vi "image_processing.vi"(5 "NG_rules":T3, 7 "parameter":T2={"image imshow"=FALSE, "side length (mm)"=0.0, "side width (mm)"=0.0, "Main Range (Threshold)"={"Lower value"=73.0, "Upper value"=255.0}, "side velocity threshold"=0.0, "Sub Range (Threshold)"={"Lower value"=73.0, "Upper value"=255.0}, "close kernel size"=0.0, "open kernel size"=0.0, "side angle offest (threshold)"=0.0}, 11 "image":T1(plugin-control)) -> (0 "PASS":bool, 2 "NG code":dbl, 3 "display image":T1(plugin-control), 4 "angle offset":dbl)   [LabVIEW 2017]
uses:
  <vilib>/vision/NI_Vision_Development_Module.lvlib
panel:
  out "side width (mm)":dbl
  out "slope array":dbl[](array[numeric])
  out "max length ratio":dbl
  out "display image 3":T1(plugin-control)
  out "display image 2":T1(plugin-control)
  out "side angle offest":dbl
  out "side length (mm)":dbl
  out "ratio (cutting offest)":dbl
  out "damaged (mil)":dbl
  out "glitch (mil)":dbl
  out "open kernel size":dbl
  out "close kernel size":dbl
  in  "side velocity threshold":dbl
  out "Main Range (Threshold)":cluster{"Lower value":sgl, "Upper value":sgl}={"Lower value"=73.0, "Upper value"=255.0}
  out "image imshow":bool
  out "time image processing":u32
  out "time load image":u32
  out "Y Resolution":i32
  out "X Resolution":i32
  out "black image":T1(plugin-control)
  out "buffer image":T1(plugin-control)
  out "Sub Range (Threshold)":cluster{"Lower value":sgl, "Upper value":sgl}={"Lower value"=73.0, "Upper value"=255.0}
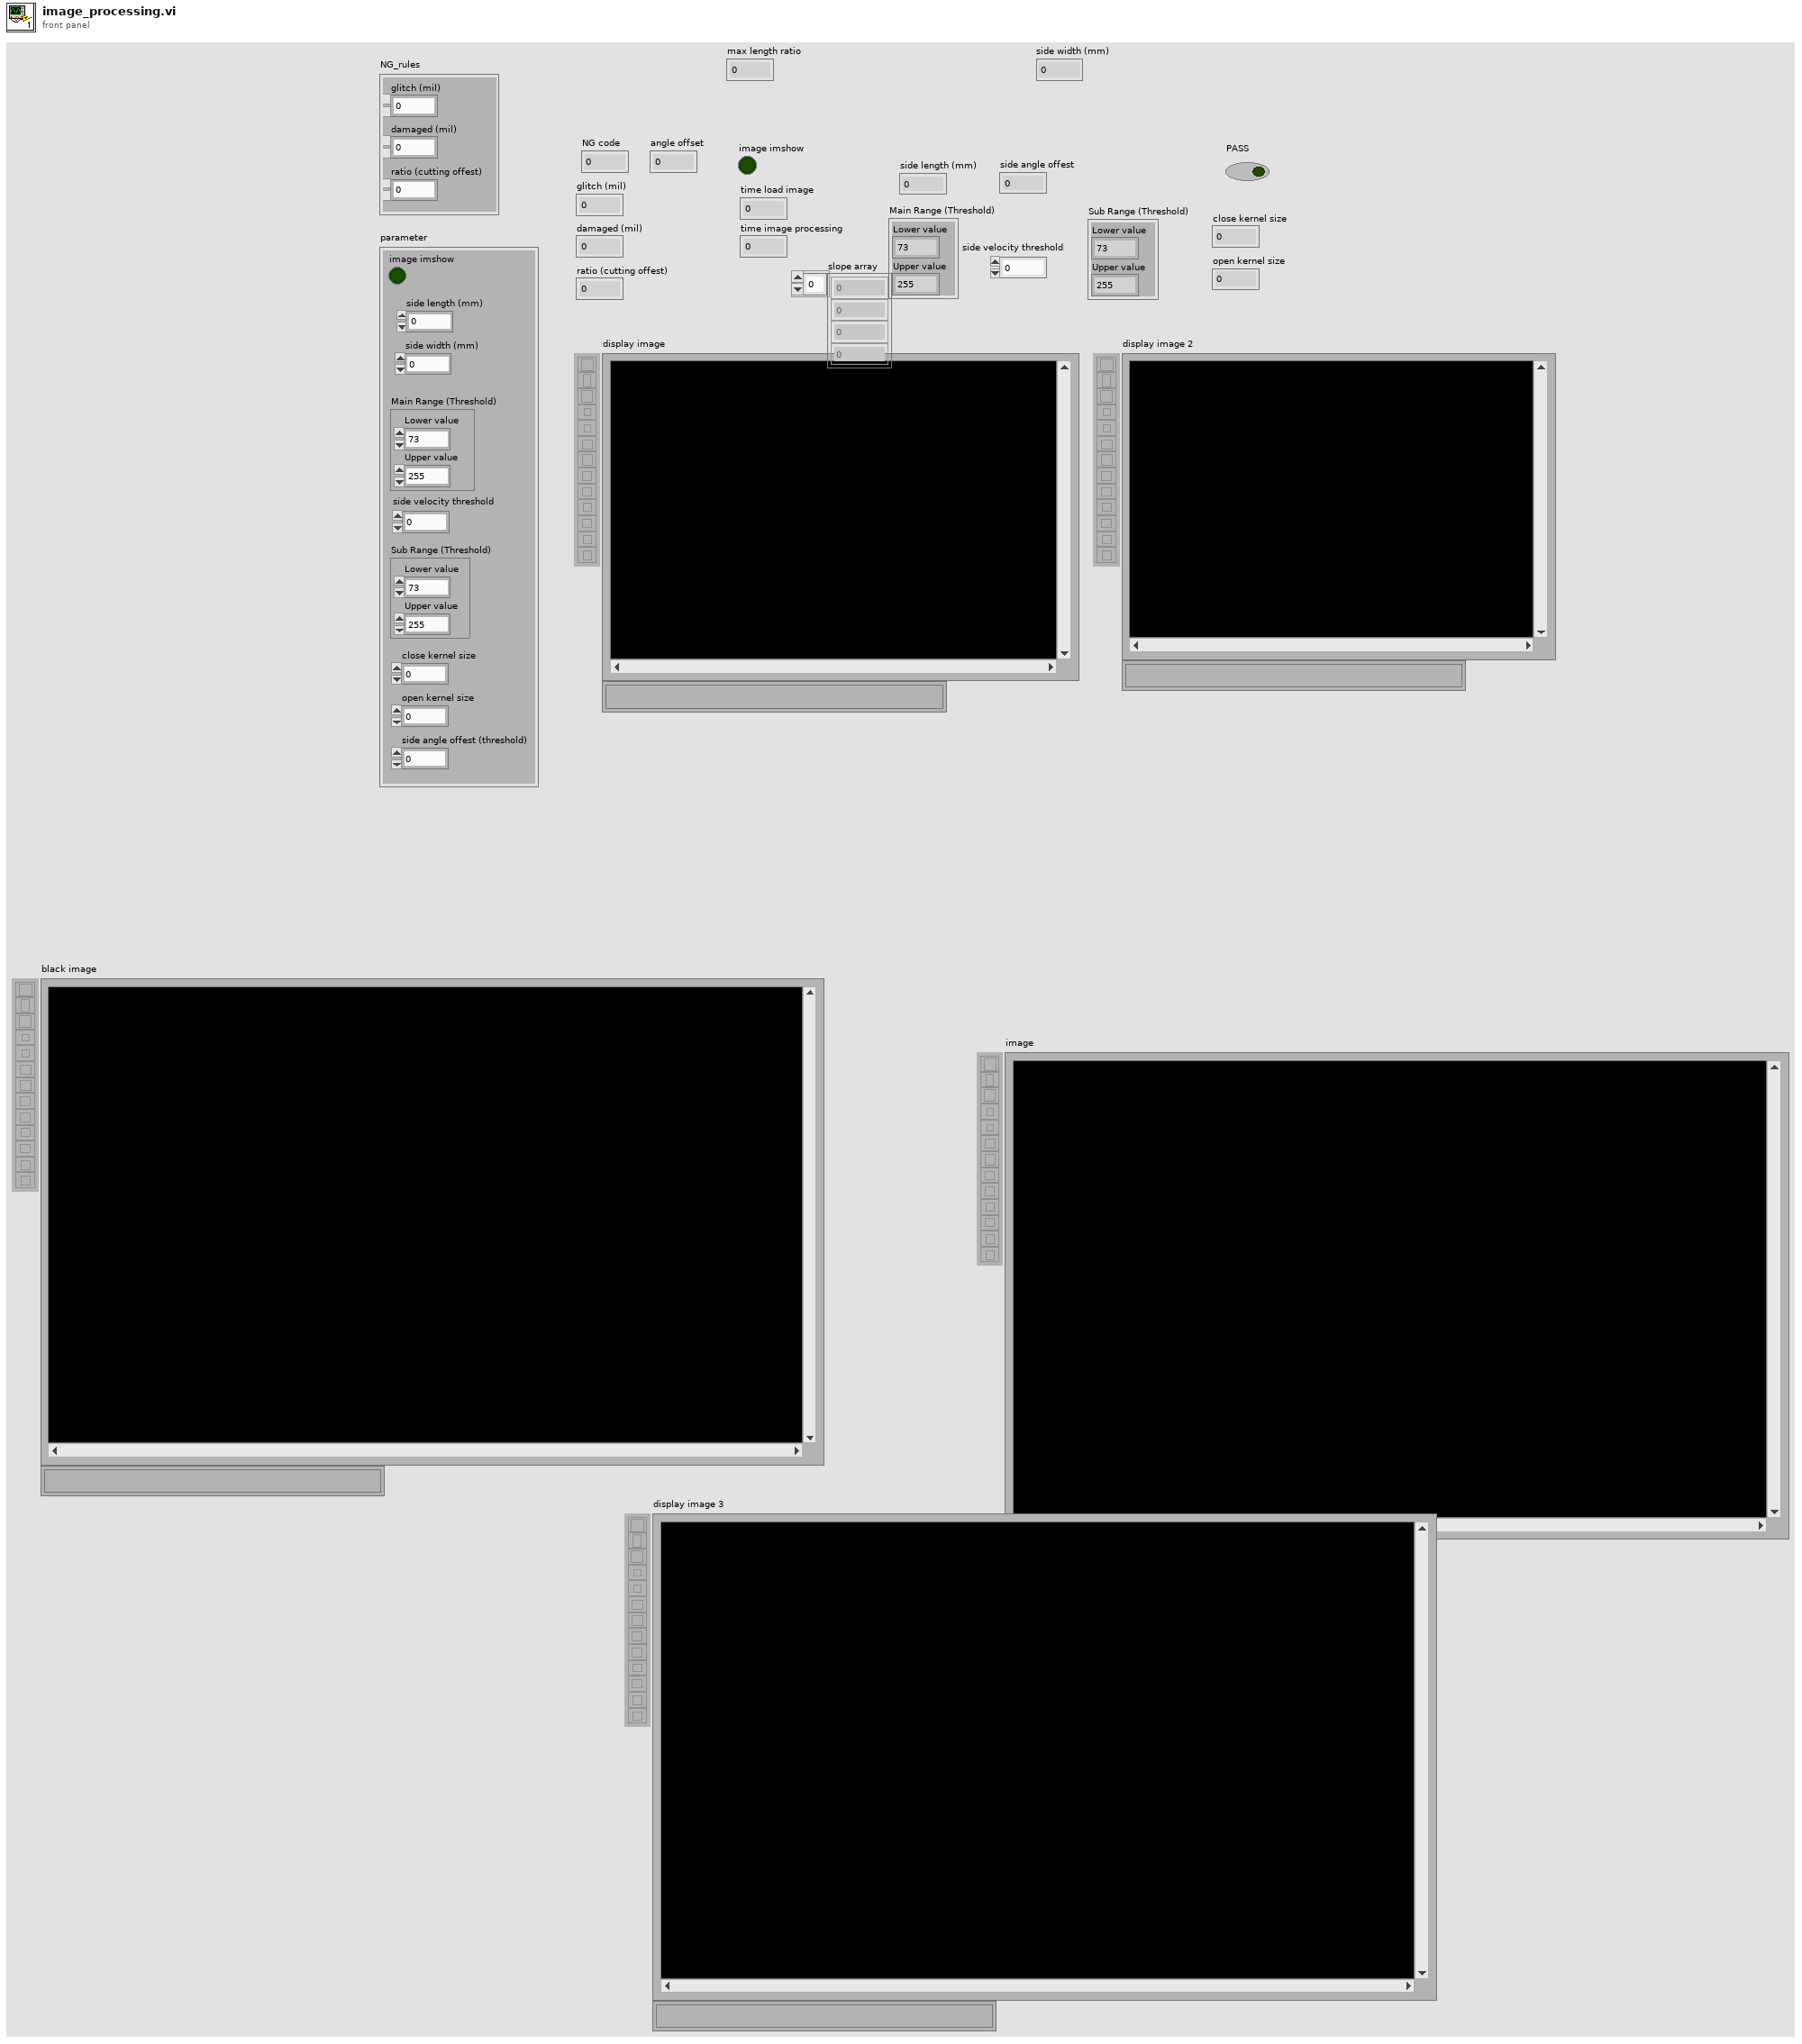
[diagram p1: front panel]
types:
  T1 = typedef "IMAQ Image.ctl" = refnum<image>
  T2 = cluster{"image imshow":bool, "side length (mm)":dbl, "side width (mm)":dbl, "Main Range (Threshold)":cluster{"Lower value":sgl, "Upper value":sgl}, "side velocity threshold":dbl, "Sub Range (Threshold)":cluster{"Lower value":sgl, "Upper value":sgl}, "close kernel size":dbl, "open kernel size":dbl, "side angle offest (threshold)":dbl}
  T3 = cluster{"glitch (mil)":dbl, "damaged (mil)":dbl, "ratio (cutting offest)":dbl}
  T4 = cluster{"Desired Font (Application)":enum16{"User-specified Font", "Application Font", "System Font", "Dialog Font"}, "[User-specified Font]":cluster{"Font Name":string, "Size":i16, "Strikeout?":bool, "Italic?":bool, "Underline?":bool, "Outline?":bool, "Shadow?":bool, "Bold?":bool, "Rotation Angle":dbl}, "Horizontal Alignment":i16, "Vertical Alignment":i16}
  T5 = enum32{"AutoM", "Close", "Dilate", "Erode", "Gradient", "Gradient out", "Gradient in", "Hit miss", "Open", "PClose", "POpen", "Thick", "Thin"}
  T6 = cluster{"Sigma":sgl, "HThresh":sgl, "LThres":sgl, "WindowSize":i32}
  T7 = cluster{"Number of Points":i32, "Open/Closed":i32, "Weight":dbl, "Contour Points":cluster{"X":dbl, "Y":dbl, "Curvature":dbl, "X Displacement":dbl, "Y Displacement":dbl}[]}[]
  T8 = cluster{"Left":i32, "Top":i32, "Right":i32, "Bottom":i32}
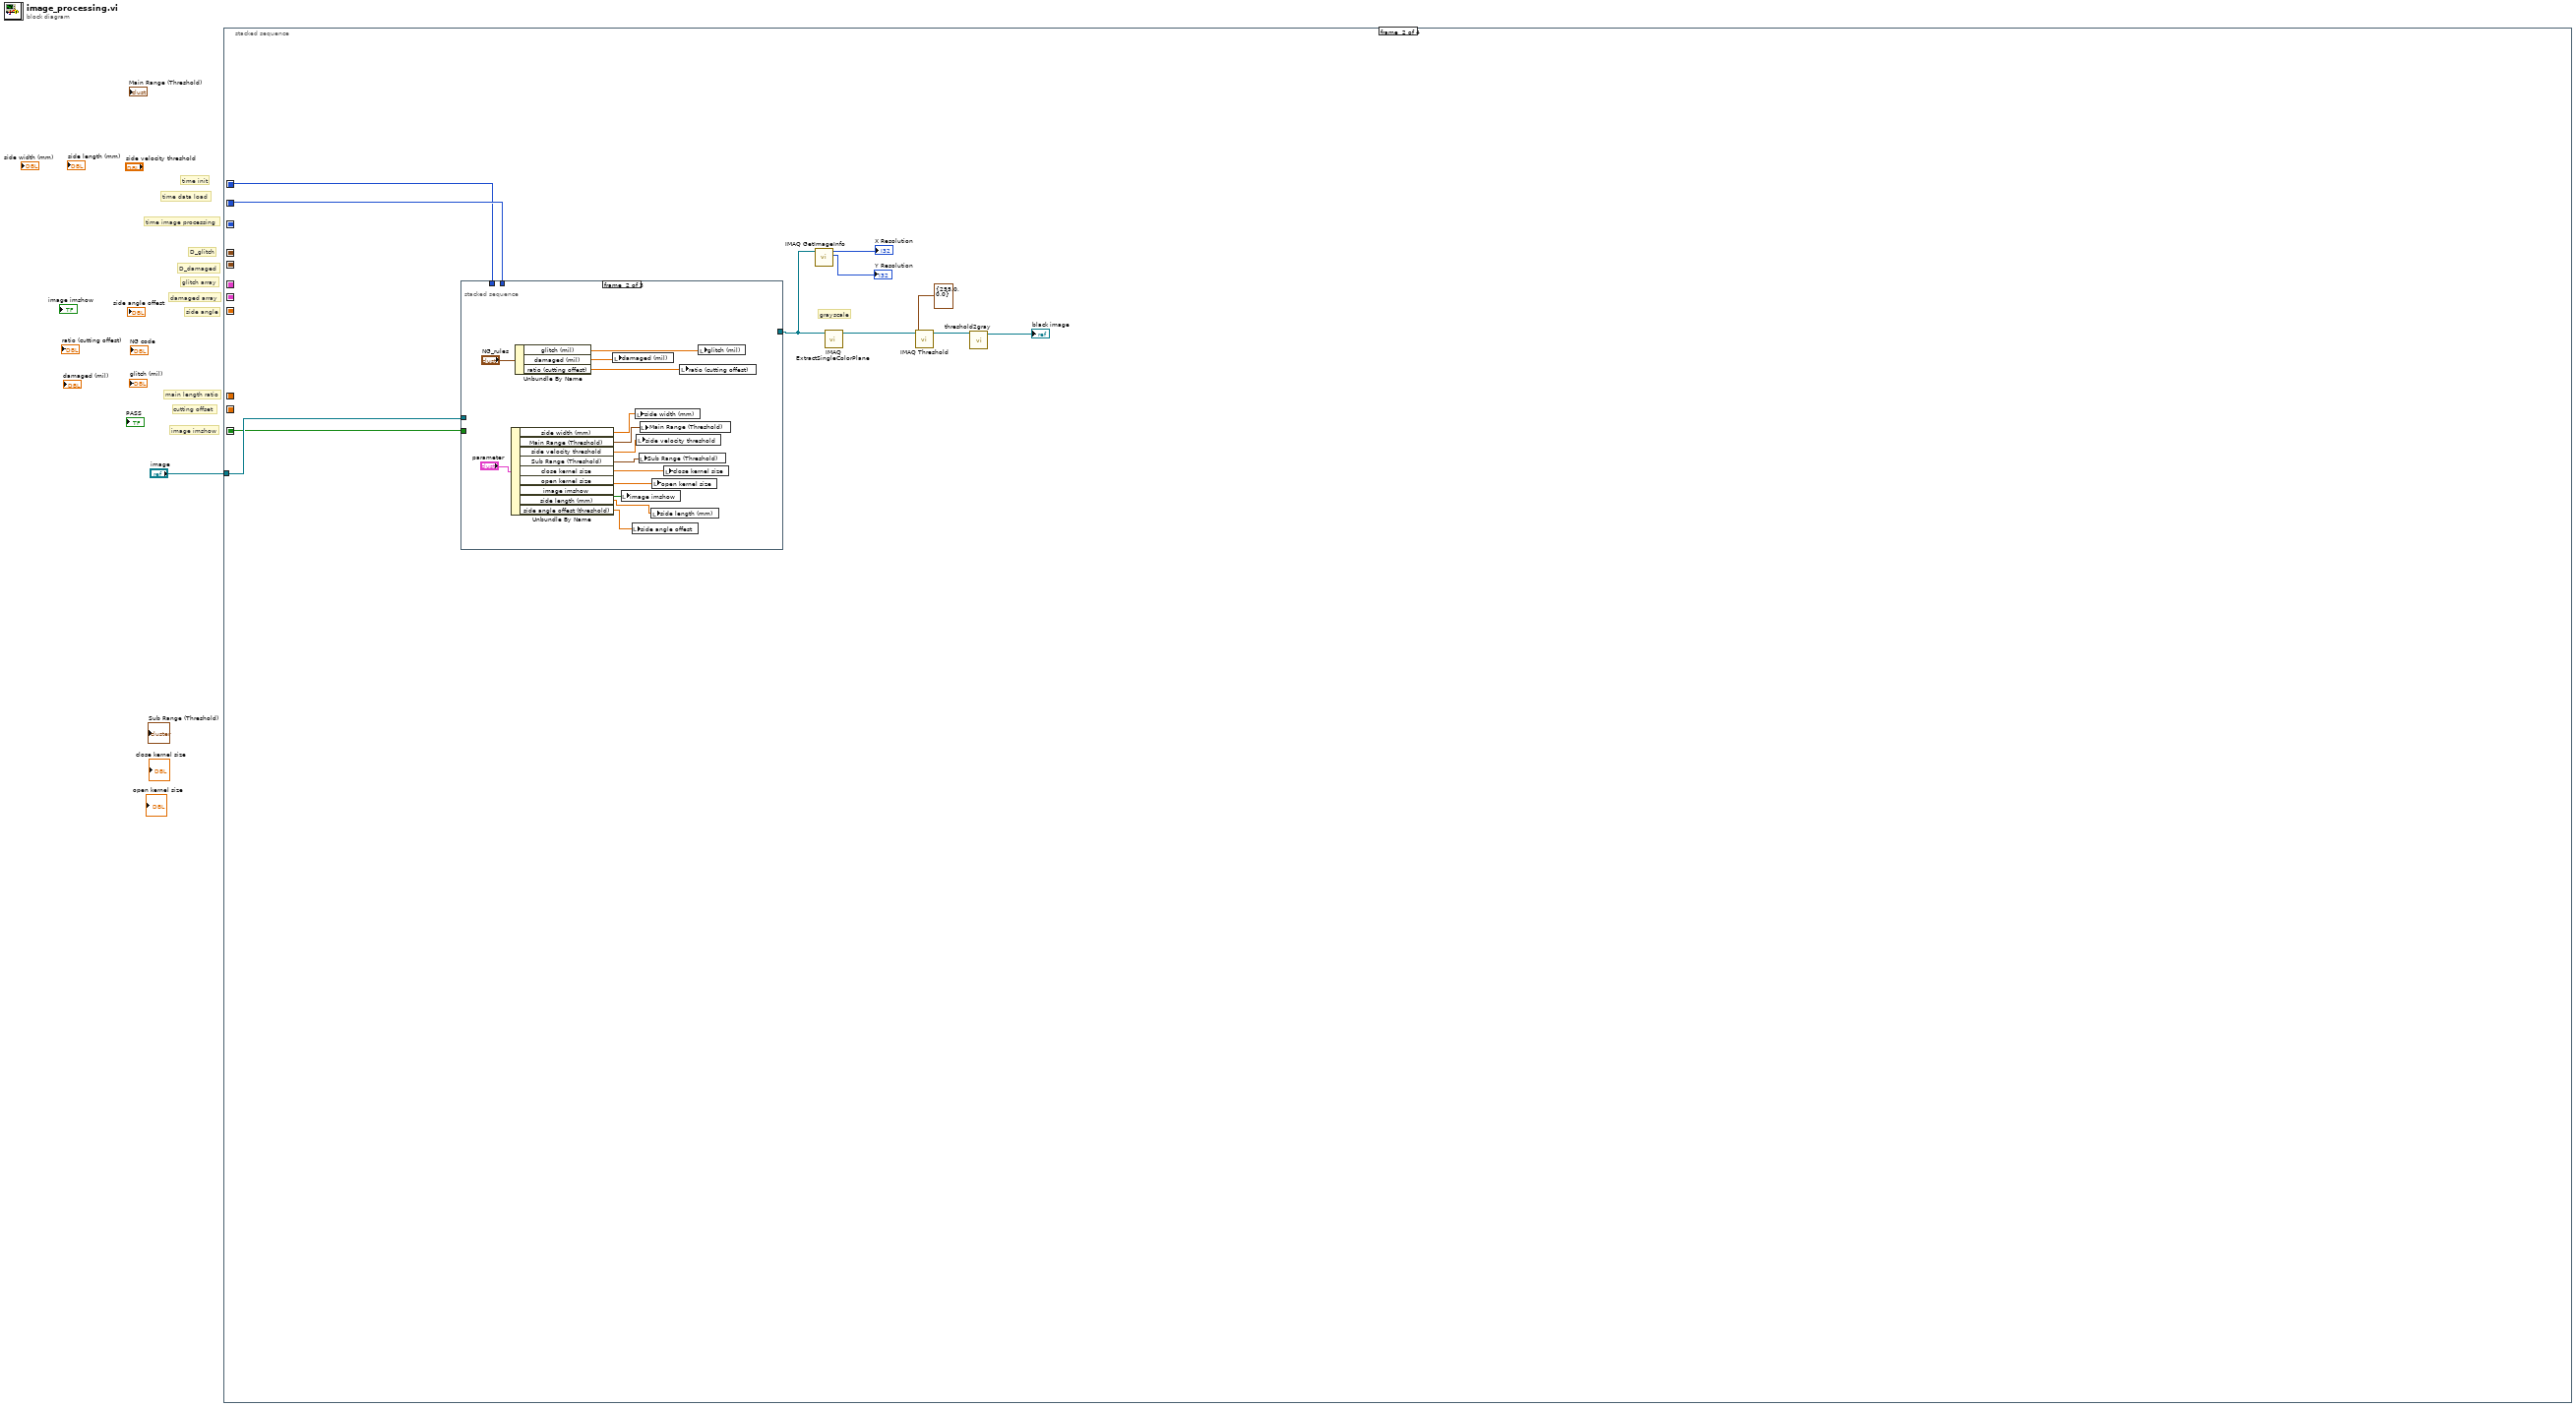
[diagram p0: block diagram]
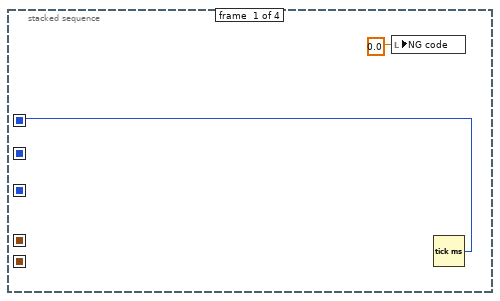
[diagram p2: hidden frame]
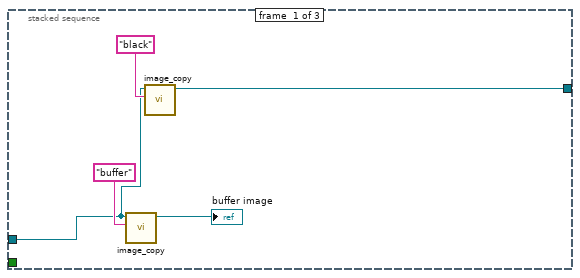
[diagram p3: hidden frame]
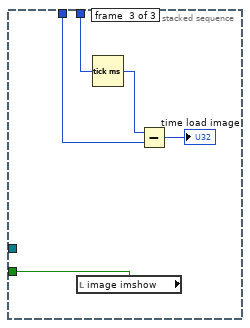
[diagram p4: hidden frame]
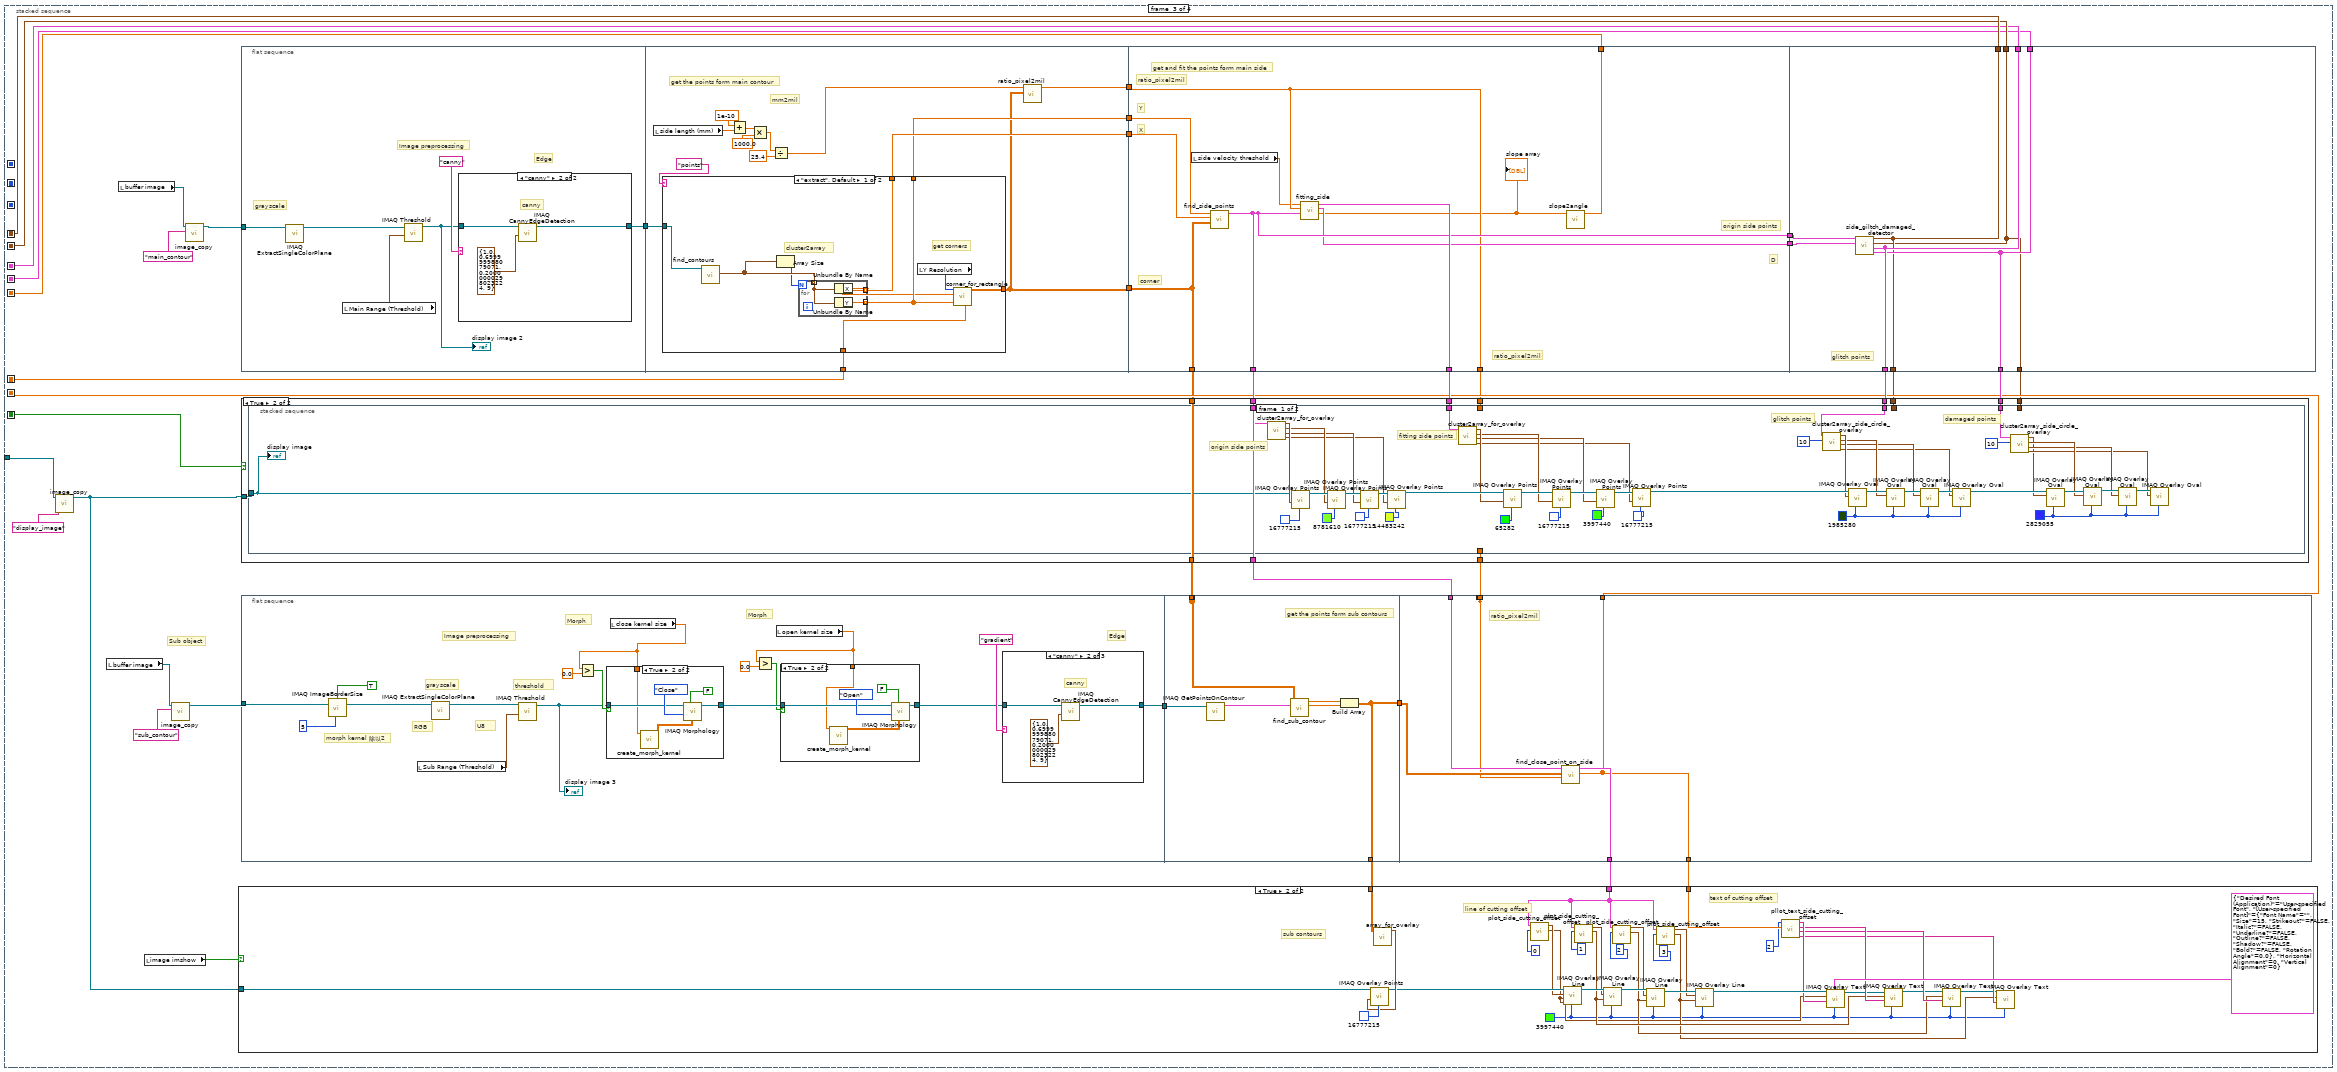
[diagram p5: hidden frame]
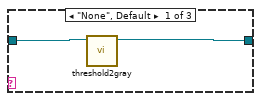
[diagram p9: hidden frame]
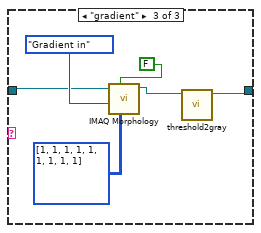
[diagram p10: hidden frame]
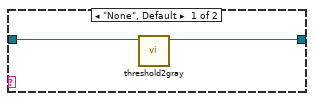
[diagram p11: hidden frame]
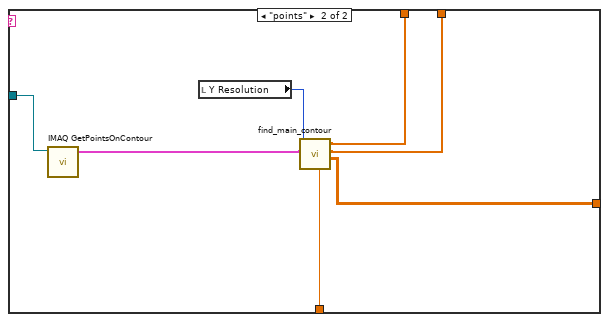
[diagram p12: hidden frame]
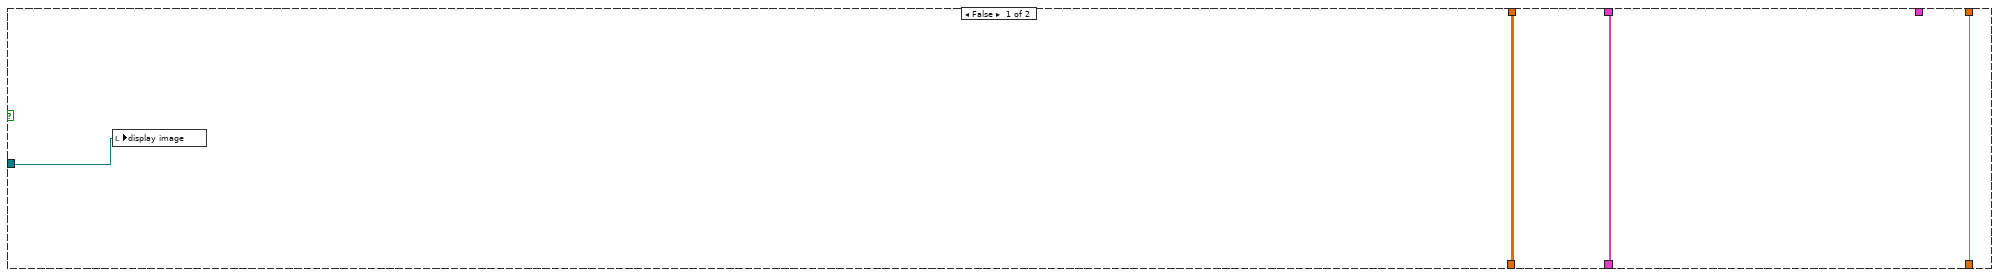
[diagram p13: hidden frame]
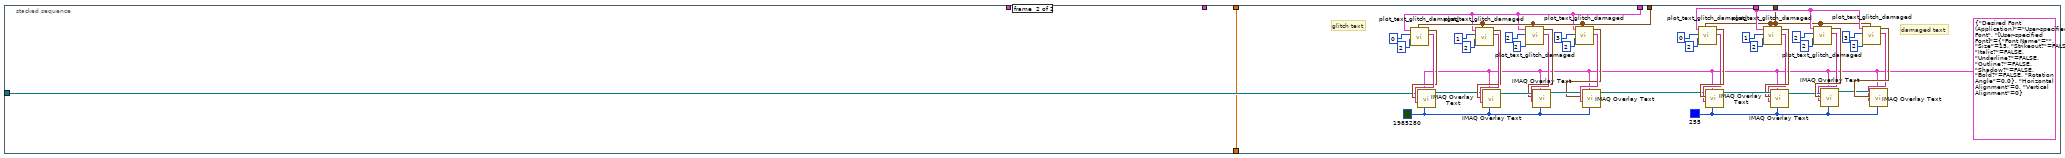
[diagram p14: hidden frame]
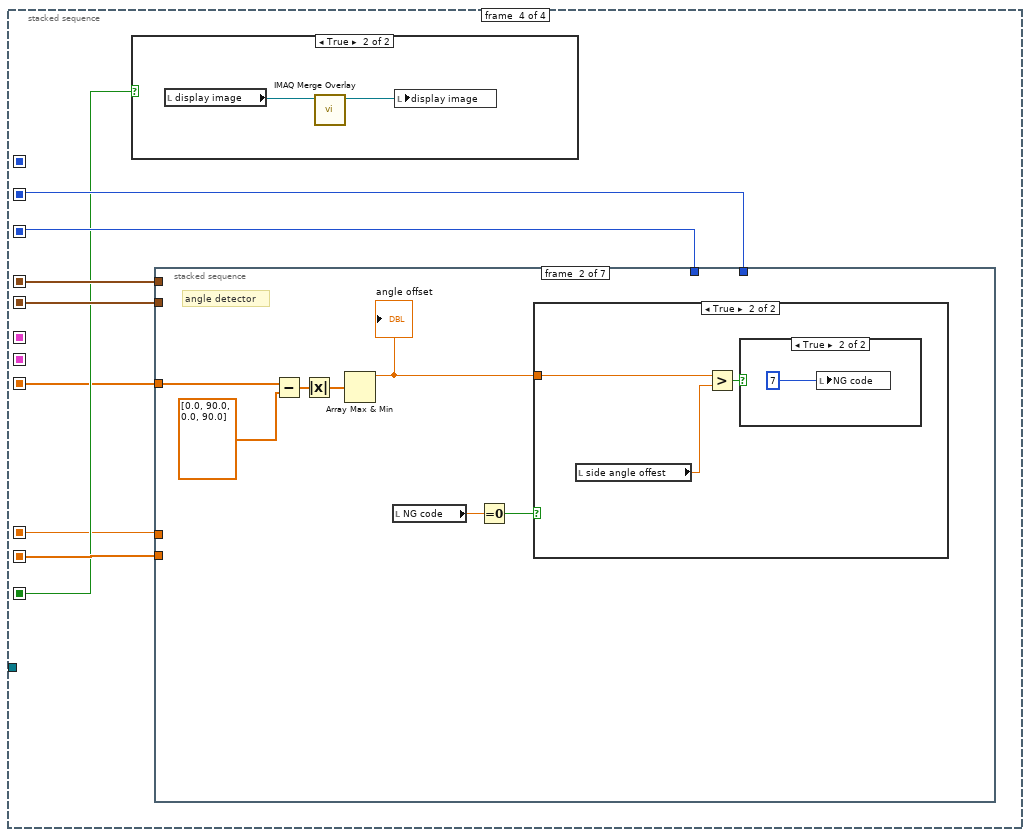
[diagram p15: hidden frame]
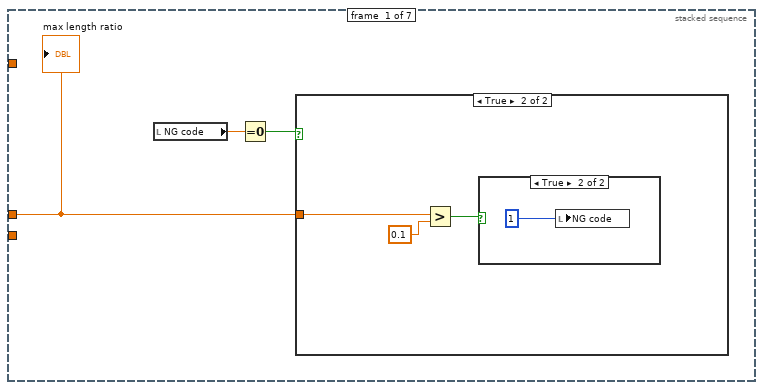
[diagram p17: hidden frame]
diagram:
  # "main length ratio"
  # "side angle"
  # "image imshow"
  # "cutting offset"
  # "damaged array"
  # "glitch array"
  # "D_damaged"
  # "D_glitch"
  # "time image processing"
  # "time data load"
  # "time init"
  n1 = stacked-sequence {
    seq-local: [w3 _ _ _] -> [_ w7 _ _]
    seq-local: [_ w8 _ _] -> [_ _ _ w340]
    seq-local: [_ _ _ w341] -> [_ _ _ _]
    seq-local: [_ _ w53 _] -> [_ _ _ w339]
    seq-local: [_ _ w52 _] -> [_ _ _ w338]
    seq-local: [_ _ w51 _] -> [_ _ _ _]
    seq-local: [_ _ w50 _] -> [_ _ _ _]
    seq-local: [_ _ w48 _] -> [_ _ _ w337]
    seq-local: [_ w4 _ _] -> [_ _ w42 w336]
    seq-local: [_ _ w41 _] -> [_ _ _ w335]
    seq-local: [_ _ w38 _] -> [_ _ _ w334]
    tunnel: "image" -> [_ w9 w60 _]
    frame #0 {
      n2 = local write "NG code"(0.0 ("NG code")) -> ()
      n3 = Tick Count (ms)() -> (millisecond timer value=w3:u32)
    }
    frame #1 {
      # "grayscale"
      n4 = stacked-sequence {
        tunnel: [w17 _ _] -> w12
        tunnel: w9 -> [w16 _ _]
        tunnel: [_ _ w37] -> w8
        tunnel: w7 -> [_ _ w36]
        tunnel: [_ _ w34] -> w4
        frame #0 {
          n5 = call "image_copy.vi"("buffer name"="buffer" ("Image Name"), "image in"=w16) -> ("imgae out"=→"buffer image":T1)  [unwired: 9 in]
          n6 = call "image_copy.vi"("buffer name"="black" ("Image Name"), "image in"=w16) -> ("imgae out"=w17:T1)  [unwired: 9 in]
        }
        frame #1 {
          n7 = Unbundle By Name("parameter") -> ("side width (mm)"=w20:dbl, "Main Range (Threshold)"=w28:cluster{"Lower value":sgl, "Upper value":sgl}, "side velocity threshold"=w27:dbl, "Sub Range (Threshold)"=w26:cluster{"Lower value":sgl, "Upper value":sgl}, "close kernel size"=w25:dbl, "open kernel size"=w24:dbl, "image imshow"=w23:bool, "side length (mm)"=w22:dbl, "side angle offest (threshold)"=w21:dbl)
          n8 = Unbundle By Name("NG_rules") -> ("glitch (mil)"=w32:dbl, "damaged (mil)"=w31:dbl, "ratio (cutting offest)"=w30:dbl)
          n9 = local write "damaged (mil)"(w31) -> ()
          n10 = local write "image imshow"(w23) -> ()
          n11 = local write "side angle offest"(w21) -> ()
          n12 = local write "side width (mm)"(w20) -> ()
          n13 = local write "side velocity threshold"(w27) -> ()
          n14 = local write "Sub Range (Threshold)"(w26) -> ()
          n15 = local write "Main Range (Threshold)"(w28) -> ()
          n16 = local write "side length (mm)"(w22) -> ()
          n17 = local write "open kernel size"(w24) -> ()
          n18 = local write "close kernel size"(w25) -> ()
          n19 = local write "ratio (cutting offest)"(w30) -> ()
          n20 = local write "glitch (mil)"(w32) -> ()
        }
        frame #2 {
          n21 = local read "image imshow"() -> (w34:bool)
          n22 = Tick Count (ms)() -> (millisecond timer value=w37:u32)
          n23 = Subtract(x=w37, y=w36) -> (x-y=→"time load image":u32)
        }
      }
      n24 = call "IMAQ GetImageInfo"("Image"=w12) -> ("Y Resolution"=→"Y Resolution":i32, "X Resolution"=→"X Resolution":i32)  [unwired: 3 in, 6 out]
      n25 = call "IMAQ ExtractSingleColorPlane"("Image Src"=w12) -> ("Image Dst Out"=w14:T1)  [unwired: 3 in, 7 out]
      n26 = call "IMAQ Threshold"("Range"=cluster{"Lower value":sgl, "Upper value":sgl} {"Lower value"=255.0, "Upper value"=0.0}, "Image Src"=w14) -> ("Image Dst Out"=w6:T1)  [unwired: 4 in, 5 out]
      n27 = call "threshold2gray.vi"("threshold image"=w6) -> ("grayscale image"=→"black image":T1)  [unwired: 10 in]
    }
    frame #2 {
      # "Sub object"
      n28 = call "image_copy.vi"("buffer name"="display_image" ("Image Name"), "image in"=w60) -> ("imgae out"=w59:T1)  [unwired: 9 in]
      n29 = local read "buffer image"() -> (w69:T1)
      n30 = local read "buffer image"() -> (w77:T1)
      n31 = local read "image imshow"() -> (w56:bool)
      n32 = call "image_copy.vi"("buffer name"="sub_contour" ("Image Name"), "image in"=w69) -> ("imgae out"=w68:T1)  [unwired: 9 in]
      n33 = call "image_copy.vi"("buffer name"="main_contour" ("Image Name"), "image in"=w77) -> ("imgae out"=w76:T1)  [unwired: 9 in]
      n34 = case shown="True" w56 {
        tunnel: w59 -> [_ w79]
        tunnel: w58 -> [_ w109]
        tunnel: w57 -> [_ w101]
        tunnel: w47 -> [_ w94]
        frame False {
        }
        frame True {
          w80 = u32 3997440 ("Text Color (black)")
          # "text of cutting offset"
          # "line of cutting offset"
          # "sub contours"
          n35 = call "array_for_overlay.vi"("Array in"=w109) -> ("Array out"=w110:cluster{"X":i32, "Y":i32}[])  [unwired: 10 in]
          n36 = call "IMAQ Overlay Points"("Color"=u32 16777215, "Array of Points"=w110, "Image"=w79) -> ("Image Out"=w108:T1)  [unwired: 7 in, 1 out]
          n37 = call "plot_side_cutting_offset.vi"("index"=0, "coord cluster"=w101) -> ("End Point out"=w81:cluster{"X":i32, "Y":i32}, "Start Point out"=w91:cluster{"X":i32, "Y":i32})  [unwired: 8 in]
          n38 = call "IMAQ Overlay Line"("Color"=w80, "End Point"=w81, "Start Point"=w91, "Image"=w108) -> ("Image Out"=w107:T1)  [unwired: 6 in, 1 out]
          n39 = call "plot_side_cutting_offset.vi"("index"=1, "coord cluster"=w101) -> ("End Point out"=w84:cluster{"X":i32, "Y":i32}, "Start Point out"=w96:cluster{"X":i32, "Y":i32})  [unwired: 8 in]
          n40 = call "IMAQ Overlay Line"("Color"=w80, "End Point"=w84, "Start Point"=w96, "Image"=w107) -> ("Image Out"=w106:T1)  [unwired: 6 in, 1 out]
          n41 = call "plot_side_cutting_offset.vi"("index"=2, "coord cluster"=w101) -> ("End Point out"=w83:cluster{"X":i32, "Y":i32}, "Start Point out"=w97:cluster{"X":i32, "Y":i32})  [unwired: 8 in]
          n42 = call "IMAQ Overlay Line"("Color"=w80, "End Point"=w83, "Start Point"=w97, "Image"=w106) -> ("Image Out"=w105:T1)  [unwired: 6 in, 1 out]
          n43 = call "plot_side_cutting_offset.vi"("index"=3, "coord cluster"=w101) -> ("End Point out"=w82:cluster{"X":i32, "Y":i32}, "Start Point out"=w98:cluster{"X":i32, "Y":i32})  [unwired: 8 in]
          n44 = call "IMAQ Overlay Line"("Color"=w80, "End Point"=w82, "Start Point"=w98, "Image"=w105) -> ("Image Out"=w99:T1)  [unwired: 6 in, 1 out]
          n45 = call "pllot_text_side_cutting_offset.vi"("D cutting offset array"=w94, "precision"=2 ("index")) -> ("Left side length"=w88:string, "Bottom side length"=w89:string, "Right side length"=w90:string, "Top side length"=w92:string)  [unwired: 6 in]
          n46 = call "IMAQ Overlay Text"("Text Color (black)"=w80, "Font, Size & Style"=T4 {"Desired Font (Application)"=enum."User-specified Font", "[User-specified Font]"={"Font Name"="", "Size"=15, "Strikeout?"=FALSE, "Italic?"=FALSE, "Underline?"=FALSE, "Outline?"=FALSE, "Shadow?"=FALSE, "Bold?"=FALSE, "Rotation Angle"=0.0}, "Horizontal Alignment"=0, "Vertical Alignment"=0}, "String"=w92, "Origin"=w81, "Image"=w99) -> ("Image Out"=w87:T1)  [unwired: 5 in, 1 out]
          n47 = call "IMAQ Overlay Text"("Text Color (black)"=w80, "String"=w90, "Origin"=w84, "Image"=w87) -> ("Image Out"=w86:T1)  [unwired: 6 in, 1 out]
          n48 = call "IMAQ Overlay Text"("Text Color (black)"=w80, "String"=w89, "Origin"=w83, "Image"=w86) -> ("Image Out"=w85:T1)  [unwired: 6 in, 1 out]
          n49 = call "IMAQ Overlay Text"("Text Color (black)"=w80, "String"=w88, "Origin"=w82, "Image"=w85) -> ()  [unwired: 6 in, 2 out]
        }
      }
      n50 = flat-sequence {
        tunnel: w76 -> [w170]
        tunnel: [w169] -> w75
        tunnel: w75 -> [w177]
        tunnel: [w183] -> w74
        tunnel: [w188] -> w72
        tunnel: [w187] -> w71
        tunnel: [w181] -> w63
        tunnel: [w176] -> w38
        tunnel: w74 -> [w208]
        tunnel: [w214] -> w73
        tunnel: w72 -> [w217]
        tunnel: w71 -> [w216]
        tunnel: [w215] -> w66
        tunnel: w63 -> [w212]
        tunnel: [w214] -> w55
        tunnel: [w213] -> w54
        tunnel: [w212] -> w44
        tunnel: [w209] -> w41
        tunnel: [w208] -> w40
        tunnel: [w221] -> w65
        tunnel: [w220] -> w64
        tunnel: w55 -> [w223]
        tunnel: w54 -> [w222]
        tunnel: [w221] -> w51
        tunnel: [w220] -> w50
        tunnel: [w219] -> w53
        tunnel: [w218] -> w52
        tunnel: [w219] -> w46
        tunnel: [w218] -> w45
        frame #0 {
          # "Image preprocessing"
          # "grayscale"
          # "Edge"
          n51 = call "IMAQ ExtractSingleColorPlane"("Image Src"=w170) -> ("Image Dst Out"=w166:T1)  [unwired: 3 in, 7 out]
          n52 = local read "Main Range (Threshold)"() -> (w167:cluster{"Lower value":sgl, "Upper value":sgl})
          n53 = call "IMAQ Threshold"("Range"=w167, "Image Src"=w166) -> ("Image Dst Out"=w165:T1)  [unwired: 4 in, 5 out]
          "display image 2" <- w165
          n54 = case shown="\"canny\"" "canny" {
            tunnel: [w171 w175] -> w169
            tunnel: w165 -> [w172 w174]
            frame "None", Default {
              n55 = call "threshold2gray.vi"("threshold image"=w172) -> ("grayscale image"=w171:T1)  [unwired: 10 in]
            }
            frame "canny" {
              # "canny"
              n56 = call "IMAQ CannyEdgeDetection"("Image Src"=w174, "Filter Parameters"=T6 {"Sigma"=1.0, "HThresh"=0.7, "LThres"=0.2, "WindowSize"=9}) -> ("Image Dst Out"=w175:T1)  [unwired: 2 in, 5 out]
            }
          }
        }
        frame #1 {
          # "mm2mil"
          # "get the points form main contour"
          n57 = local read "side length (mm)"() -> (w178:dbl)
          n58 = case shown="\"extract\", Default" "points" {
            tunnel: w177 -> [w193 w207]
            tunnel: [w194 w202] -> w183
            tunnel: [w192 w203] -> w187
            tunnel: [w191 w204] -> w188
            tunnel: [w190 w201] -> w176
            frame "extract", Default {
              # "get corners"
              # "cluster2array"
              n59 = call "find_contours.vi"("image in"=w193) -> ("Source Image Points"=w197:cluster{"X":dbl, "Y":dbl}[])  [unwired: 9 in, 1 out]
              n60 = Array Size(array=w197) -> (size(s)=w195:i32)
              n61 = for {
                N: w195 -> [_]
                tunnel: w197 -> [w199] mode=indexing
                tunnel: [w200] -> w191 mode=indexing
                tunnel: [w198] -> w192 mode=indexing
                n62 = Unbundle By Name(w199) -> ("X"=w200:dbl)
                n63 = Unbundle By Name(w199) -> ("Y"=w198:dbl)
              }
              n64 = local read "Y Resolution"() -> (w196:i32)
              n65 = call "corner_for_rectangle.vi"("Y"=w192, "X"=w191, "Y Resolution"=w196) -> ("corner"=w194:dbl[][], "length ratio"=w190:dbl)  [unwired: 6 in, 1 out]
            }
            frame "points" {
              n66 = call "IMAQ GetPointsOnContour"("Image (Edge Image)"=w207) -> ("Segment Information"=w205:T7)  [unwired: 3 in, 2 out]
              n67 = local read "Y Resolution"() -> (w206:i32)
              n68 = call "find_main_contour.vi"("Segment Information"=w205, "Y Resolution"=w206) -> ("max corner"=w202:dbl[][], "Y"=w203:dbl[], "X"=w204:dbl[], "max length ratio"=w201:dbl)  [unwired: 6 in]
            }
          }
          n69 = Add(x=1e-10, y=w178) -> (x+y=w179:dbl)
          n70 = Multiply(x=w179, y=1000.0) -> (x*y=w185:dbl)
          n71 = Divide(x=w185, y=25.4) -> (x/y=w182:dbl)
          n72 = call "ratio_pixel2mil.vi"("max corner in"=w183, "side length (mm)"=w182) -> ("ratio"=w181:dbl)  [unwired: 9 in]
        }
        frame #2 {
          # "ratio_pixel2mil"
          # "origin side points"
          # "D"
          # "corner"
          # "X"
          # "Y"
          # "ratio_pixel2mil"
          # "get and fit the points form main side"
          n73 = local read "side velocity threshold"() -> (w211:dbl)
          n74 = call "find_side_points.vi"("corner"=w208, "X  coords array"=w217, "Y coords array"=w216) -> ("side of clusters"=w214:cluster{"Array out":dbl[][]}[])  [unwired: 8 in]
          n75 = call "fitting_side.vi"("side of clusters"=w214, "ratio"=w212, "side velocity threshold"=w211) -> ("slope array"=w210:dbl[], "D of clusters"=w213:cluster{"D":ext[]}[], "fitting clusters"=w215:cluster{"fitting array":dbl[][]}[])  [unwired: 6 in]
          "slope array" <- w210
          n76 = call "slope2angle.vi"("slope array"=w210) -> ("x/y"=w209:dbl[])  [unwired: 10 in]
        }
        frame #3 {
          # "glitch points"
          n77 = call "side_giltch_damaged_detector.vi"("D of clusters"=w222, "side of clusters"=w223) -> ("damaged clusters"=w220:cluster{"damaged coord":dbl[]}[], "giltch of clusters"=w221:cluster{"giltch_coord":dbl[]}[], "D damaged of clusters"=w218:cluster{"D_damaged":ext}[], "D giltch of clusters"=w219:cluster{"D_giltch":ext}[])  [unwired: 6 in]
        }
      }
      n78 = flat-sequence {
        tunnel: w68 -> [w126]
        tunnel: [w122] -> w67
        tunnel: w67 -> [w159]
        tunnel: [w155] -> w62
        tunnel: [w155] -> w58
        tunnel: [w154] -> _
        tunnel: w39 -> [w154]
        tunnel: w62 -> [w164]
        tunnel: [w163] -> w57
        tunnel: w49 -> [w162]
        tunnel: [w160] -> w48
        tunnel: [w160] -> w47
        tunnel: [w161] -> _
        tunnel: w43 -> [w161]
        frame #0 {
          # "Morph"
          # "Image preprocessing"
          # "Morph"
          # "morph kernel 除以2"
          # "Edge"
          # "U8"
          # "RGB"
          # "threshold"
          # "grayscale"
          n79 = call "IMAQ ImageBorderSize"("Get/Set Status? (Set)"=TRUE, "Image"=w126, "Image border size in"=5) -> ("Image Out"=w125:T1)  [unwired: 1 in, 2 out]
          n80 = local read "Sub Range (Threshold)"() -> (w115:cluster{"Lower value":sgl, "Upper value":sgl})
          n81 = call "IMAQ ExtractSingleColorPlane"("Image Src"=w125) -> ("Image Dst Out"=w128:T1)  [unwired: 3 in, 7 out]
          n82 = call "IMAQ Threshold"("Range"=w115, "Image Src"=w128) -> ("Image Dst Out"=w112:T1)  [unwired: 4 in, 5 out]
          "display image 3" <- w112
          n83 = local read "close kernel size"() -> (w114:dbl)
          n84 = Greater?(x=w114, y=0.0) -> (0:w119:bool)
          n85 = case shown="True" w119 {
            tunnel: w112 -> [w136 w141]
            tunnel: [w136 w140] -> w120
            tunnel: w114 -> [_ w139]
            frame False {
            }
            frame True {
              n86 = call "create_morph_kernel.vi"("kernel size"=w139) -> ("kernel"=w138:dbl[][])  [unwired: 10 in]
              n87 = call "IMAQ Morphology"("Structuring Element"=w138, "Square/Hexa (Square)"=FALSE, "Operation"=T5."Close", "Image Src"=w141) -> ("Image Dst Out"=w140:T1)  [unwired: 3 in, 4 out]
            }
          }
          n88 = local read "open kernel size"() -> (w113:dbl)
          n89 = Greater?(x=w113, y=0.0) -> (0:w116:bool)
          n90 = case shown="True" w116 {
            tunnel: [w129 w134] -> w121
            tunnel: w120 -> [w129 w133]
            tunnel: w113 -> [_ w130]
            frame False {
            }
            frame True {
              n91 = call "create_morph_kernel.vi"("kernel size"=w130) -> ("kernel"=w131:dbl[][])  [unwired: 10 in]
              n92 = call "IMAQ Morphology"("Structuring Element"=w131, "Square/Hexa (Square)"=FALSE, "Operation"=T5."Open", "Image Src"=w133) -> ("Image Dst Out"=w134:T1)  [unwired: 3 in, 4 out]
            }
          }
          n93 = case shown="\"canny\"" "gradient" {
            tunnel: [w143 w147 w148] -> w122
            tunnel: w121 -> [w144 w146 w150]
            frame "None", Default {
              n94 = call "threshold2gray.vi"("threshold image"=w144) -> ("grayscale image"=w143:T1)  [unwired: 10 in]
            }
            frame "canny" {
              # "canny"
              n95 = call "IMAQ CannyEdgeDetection"("Image Src"=w146, "Filter Parameters"=T6 {"Sigma"=1.0, "HThresh"=0.7, "LThres"=0.2, "WindowSize"=9}) -> ("Image Dst Out"=w147:T1)  [unwired: 2 in, 5 out]
            }
            frame "gradient" {
              n96 = call "IMAQ Morphology"("Structuring Element"=i32[][] [[1, 1, 1], [1, 1, 1], [1, 1, 1]], "Square/Hexa (Square)"=FALSE, "Operation"=T5."Gradient in", "Image Src"=w150) -> ("Image Dst Out"=w149:T1)  [unwired: 3 in, 4 out]
              n97 = call "threshold2gray.vi"("threshold image"=w149) -> ("grayscale image"=w148:T1)  [unwired: 10 in]
            }
          }
        }
        frame #1 {
          # "get the points form sub contours"
          n98 = call "IMAQ GetPointsOnContour"("Image (Edge Image)"=w159) -> ("Segment Information"=w158:T7)  [unwired: 3 in, 2 out]
          n99 = call "find_sub_contour.vi"("Segment Information"=w158, "rectangle corner"=w154) -> ("Y"=w156:dbl[], "X"=w157:dbl[])  [unwired: 8 in]
          n100 = Build Array(w157, w156) -> (w155:dbl[][])
        }
        frame #2 {
          # "ratio_pixel2mil"
          n101 = call "find_close_point_on_side.vi"("ratio_pixel2mil"=w161, "Array"=w164, "fitting clusters"=w162) -> ("D cutting offset array"=w160:ext[], "coord cluster"=w163:cluster{dbl[][]}[])  [unwired: 7 in]
        }
      }
      n102 = case shown="True" w42 {
        tunnel: w59 -> [w226 w237]
        tunnel: w73 -> [w225 w229]
        tunnel: w66 -> [_ w234]
        tunnel: w65 -> [_ w235]
        tunnel: w64 -> [_ w236]
        tunnel: [w225 w229] -> w49
        tunnel: w46 -> [_ w233]
        tunnel: w45 -> [_ w232]
        tunnel: w44 -> [w227 w231]
        tunnel: [w227 w230] -> w43
        tunnel: [w224 w228] -> w39
        tunnel: w40 -> [w224 w228]
        frame False {
          n103 = local write "display image"(w226) -> ()
        }
        frame True {
          n104 = stacked-sequence {
            tunnel: w237 -> [w238 w329]
            tunnel: w229 -> [w260 _]
            tunnel: w236 -> [w245 w292]
            tunnel: w235 -> [w240 w314]
            tunnel: w234 -> [w239 _]
            tunnel: w233 -> [_ w316]
            tunnel: w232 -> [_ w291]
            tunnel: w231 -> [_ w287]
            tunnel: [_ w287] -> w230
            frame #0 {
              w262 = u32 2829055 ("Color")
              w263 = u32 1985280 ("Color")
              # "damaged points"
              # "glitch points"
              # "fitting side points"
              # "origin side points"
              n105 = call "cluster2array_for_overlay.vi"("side of clusters"=w260) -> ("Left side points"=w256:cluster{"X":i32, "Y":i32}[], "Bottom side points"=w257:cluster{"X":i32, "Y":i32}[], "Right side points"=w258:cluster{"X":i32, "Y":i32}[], "Top side points"=w259:cluster{"X":i32, "Y":i32}[])  [unwired: 7 in]
              n106 = call "IMAQ Overlay Points"("Color"=u32 16777215, "Array of Points"=w259, "Image"=w238) -> ("Image Out"=w282:T1)  [unwired: 7 in, 1 out]
              n107 = call "IMAQ Overlay Points"("Color"=u32 8781610, "Array of Points"=w258, "Image"=w282) -> ("Image Out"=w284:T1)  [unwired: 7 in, 1 out]
              n108 = call "IMAQ Overlay Points"("Color"=u32 16777215, "Array of Points"=w257, "Image"=w284) -> ("Image Out"=w283:T1)  [unwired: 7 in, 1 out]
              n109 = call "IMAQ Overlay Points"("Color"=u32 14483242, "Array of Points"=w256, "Image"=w283) -> ("Image Out"=w271:T1)  [unwired: 7 in, 1 out]
              n110 = call "cluster2array_for_overlay.vi"("side of clusters"=w239) -> ("Left side points"=w252:cluster{"X":i32, "Y":i32}[], "Bottom side points"=w253:cluster{"X":i32, "Y":i32}[], "Right side points"=w254:cluster{"X":i32, "Y":i32}[], "Top side points"=w255:cluster{"X":i32, "Y":i32}[])  [unwired: 7 in]
              n111 = call "IMAQ Overlay Points"("Color"=u32 65282, "Array of Points"=w255, "Image"=w271) -> ("Image Out"=w275:T1)  [unwired: 7 in, 1 out]
              n112 = call "IMAQ Overlay Points"("Color"=u32 16777215, "Array of Points"=w254, "Image"=w275) -> ("Image Out"=w273:T1)  [unwired: 7 in, 1 out]
              n113 = call "IMAQ Overlay Points"("Color"=u32 3997440, "Array of Points"=w253, "Image"=w273) -> ("Image Out"=w274:T1)  [unwired: 7 in, 1 out]
              n114 = call "IMAQ Overlay Points"("Color"=u32 16777215, "Array of Points"=w252, "Image"=w274) -> ("Image Out"=w261:T1)  [unwired: 7 in, 1 out]
              n115 = call "cluster2array_side_circle_overlay.vi"("radius"=10 ("index"), "giltch of clusters"=w240) -> ("Left side points"=w248:T8, "Bottom side points"=w249:T8, "Right side points"=w250:T8, "Top side points"=w251:T8)  [unwired: 6 in]
              n116 = call "IMAQ Overlay Oval"("Color"=w263, "Bounding Rectangle"=w251, "Image"=w261) -> ("Image Out"=w270:T1)  [unwired: 7 in, 1 out]
              n117 = call "IMAQ Overlay Oval"("Color"=w263, "Bounding Rectangle"=w250, "Image"=w270) -> ("Image Out"=w269:T1)  [unwired: 7 in, 1 out]
              n118 = call "IMAQ Overlay Oval"("Color"=w263, "Bounding Rectangle"=w249, "Image"=w269) -> ("Image Out"=w268:T1)  [unwired: 7 in, 1 out]
              n119 = call "IMAQ Overlay Oval"("Color"=w263, "Bounding Rectangle"=w248, "Image"=w268) -> ("Image Out"=w264:T1)  [unwired: 7 in, 1 out]
              n120 = call "cluster2array_side_circle_overlay.vi"("radius"=10 ("index"), "giltch of clusters"=w245) -> ("Left side points"=w242:T8, "Bottom side points"=w243:T8, "Right side points"=w244:T8, "Top side points"=w241:T8)  [unwired: 6 in]
              n121 = call "IMAQ Overlay Oval"("Color"=w262, "Bounding Rectangle"=w241, "Image"=w264) -> ("Image Out"=w265:T1)  [unwired: 7 in, 1 out]
              n122 = call "IMAQ Overlay Oval"("Color"=w262, "Bounding Rectangle"=w244, "Image"=w265) -> ("Image Out"=w266:T1)  [unwired: 7 in, 1 out]
              n123 = call "IMAQ Overlay Oval"("Color"=w262, "Bounding Rectangle"=w243, "Image"=w266) -> ("Image Out"=w267:T1)  [unwired: 7 in, 1 out]
              n124 = call "IMAQ Overlay Oval"("Color"=w262, "Bounding Rectangle"=w242, "Image"=w267) -> ()  [unwired: 7 in, 2 out]
              "display image" <- w238
            }
            frame #1 {
              w286 = u32 1985280 ("Color")
              w289 = u32 255 ("Text Color (black)")
              w290 = T4 {"Desired Font (Application)"=enum."User-specified Font", "[User-specified Font]"={"Font Name"="", "Size"=15, "Strikeout?"=FALSE, "Italic?"=FALSE, "Underline?"=FALSE, "Outline?"=FALSE, "Shadow?"=FALSE, "Bold?"=FALSE, "Rotation Angle"=0.0}, "Horizontal Alignment"=0, "Vertical Alignment"=0} ("Font, Size & Style")
              # "damaged text"
              # "glitch text"
              n125 = call "plot_text_glitch_damaged.vi"("D of clusters"=w316, "precision"=2 ("index (page)"), "index"=0 ("index (page)"), "array clusters"=w314) -> ("string"=w331:string, "Origin"=w330:cluster{"X":i32, "Y":i32})  [unwired: 6 in]
              n126 = call "IMAQ Overlay Text"("Text Color (black)"=w286, "Font, Size & Style"=w290, "String"=w331, "Origin"=w330, "Image"=w329) -> ("Image Out"=w324:T1)  [unwired: 5 in, 1 out]
              n127 = call "plot_text_glitch_damaged.vi"("D of clusters"=w316, "precision"=2 ("index (page)"), "index"=1 ("index (page)"), "array clusters"=w314) -> ("string"=w328:string, "Origin"=w325:cluster{"X":i32, "Y":i32})  [unwired: 6 in]
              n128 = call "IMAQ Overlay Text"("Text Color (black)"=w286, "Font, Size & Style"=w290, "String"=w328, "Origin"=w325, "Image"=w324) -> ("Image Out"=w317:T1)  [unwired: 5 in, 1 out]
              n129 = call "plot_text_glitch_damaged.vi"("D of clusters"=w316, "precision"=2 ("index (page)"), "index"=2 ("index (page)"), "array clusters"=w314) -> ("string"=w321:string, "Origin"=w312:cluster{"X":i32, "Y":i32})  [unwired: 6 in]
              n130 = call "IMAQ Overlay Text"("Text Color (black)"=w286, "Font, Size & Style"=w290, "String"=w321, "Origin"=w312, "Image"=w317) -> ("Image Out"=w315:T1)  [unwired: 5 in, 1 out]
              n131 = call "plot_text_glitch_damaged.vi"("D of clusters"=w316, "precision"=2 ("index (page)"), "index"=3 ("index (page)"), "array clusters"=w314) -> ("string"=w320:string, "Origin"=w313:cluster{"X":i32, "Y":i32})  [unwired: 6 in]
              n132 = call "IMAQ Overlay Text"("Text Color (black)"=w286, "Font, Size & Style"=w290, "String"=w320, "Origin"=w313, "Image"=w315) -> ("Image Out"=w288:T1)  [unwired: 5 in, 1 out]
              n133 = call "plot_text_glitch_damaged.vi"("D of clusters"=w291, "precision"=2 ("index (page)"), "index"=0 ("index (page)"), "array clusters"=w292) -> ("string"=w295:string, "Origin"=w296:cluster{"X":i32, "Y":i32})  [unwired: 6 in]
              n134 = call "IMAQ Overlay Text"("Text Color (black)"=w289, "Font, Size & Style"=w290, "String"=w295, "Origin"=w296, "Image"=w288) -> ("Image Out"=w301:T1)  [unwired: 5 in, 1 out]
              n135 = call "plot_text_glitch_damaged.vi"("D of clusters"=w291, "precision"=2 ("index (page)"), "index"=1 ("index (page)"), "array clusters"=w292) -> ("string"=w297:string, "Origin"=w300:cluster{"X":i32, "Y":i32})  [unwired: 6 in]
              n136 = call "IMAQ Overlay Text"("Text Color (black)"=w289, "Font, Size & Style"=w290, "String"=w297, "Origin"=w300, "Image"=w301) -> ("Image Out"=w308:T1)  [unwired: 5 in, 1 out]
              n137 = call "plot_text_glitch_damaged.vi"("D of clusters"=w291, "precision"=2 ("index (page)"), "index"=2 ("index (page)"), "array clusters"=w292) -> ("string"=w304:string, "Origin"=w311:cluster{"X":i32, "Y":i32})  [unwired: 6 in]
              n138 = call "IMAQ Overlay Text"("Text Color (black)"=w289, "Font, Size & Style"=w290, "String"=w304, "Origin"=w311, "Image"=w308) -> ("Image Out"=w309:T1)  [unwired: 5 in, 1 out]
              n139 = call "plot_text_glitch_damaged.vi"("D of clusters"=w291, "precision"=2 ("index (page)"), "index"=3 ("index (page)"), "array clusters"=w292) -> ("string"=w305:string, "Origin"=w310:cluster{"X":i32, "Y":i32})  [unwired: 6 in]
              n140 = call "IMAQ Overlay Text"("Text Color (black)"=w289, "Font, Size & Style"=w290, "String"=w305, "Origin"=w310, "Image"=w309) -> ()  [unwired: 5 in, 2 out]
            }
          }
        }
      }
    }
    frame #3 {
      n141 = case shown="True" w336 {
        frame False {
        }
        frame True {
          n142 = local read "display image"() -> (w343:T1)
          n143 = call "IMAQ Merge Overlay"("Image Src"=w343) -> ("Image Dst Out"=w342:T1)  [unwired: 9 in, 1 out]
          n144 = local write "display image"(w342) -> ()
        }
      }
      n145 = stacked-sequence {
        tunnel: [_ _ _ _ _ _ w417] -> w341
        tunnel: w340 -> [_ _ _ _ _ _ w416]
        tunnel: w339 -> [_ _ w364 _ _ _ _]
        tunnel: w338 -> [_ _ _ w371 _ _ _]
        tunnel: w337 -> [_ _ _ _ w380 _ _]
        tunnel: w335 -> [_ w357 _ _ _ _ _]
        tunnel: w334 -> [w346 _ _ _ _ _ _]
        frame #0 {
          n146 = local read "NG code"() -> (w345:dbl)
          n147 = Equal To 0?(x=w345) -> (x = 0?=w344:bool)
          n148 = case shown="True" w344 {
            tunnel: w346 -> [_ w349]
            frame False {
            }
            frame True {
              n149 = Greater?(x=w349, y=0.1) -> (0:w347:bool)
              n150 = case shown="True" w347 {
                frame False {
                }
                frame True {
                  n151 = local write "NG code"(1) -> ()
                }
              }
            }
          }
          "max length ratio" <- w346
        }
        frame #1 {
          # "angle detector"
          n152 = Subtract(x=w357, y=dbl[] [0.0, 90.0, 0.0, 90.0] ("x/y")) -> (x-y=w355:dbl[])
          n153 = Absolute Value(x=w355) -> (abs(x)=w354:dbl[])
          n154 = Array Max & Min(array=w354) -> (max value=w353:dbl)  [unwired: 3 out]
          "angle offset" <- w353
          n155 = local read "NG code"() -> (w352:dbl)
          n156 = Equal To 0?(x=w352) -> (x = 0?=w351:bool)
          n157 = case shown="True" w351 {
            tunnel: w353 -> [_ w359]
            frame False {
            }
            frame True {
              n158 = local read "side angle offest"() -> (w360:dbl)
              n159 = Greater?(x=w359, y=w360) -> (0:w358:bool)
              n160 = case shown="True" w358 {
                frame False {
                }
                frame True {
                  n161 = local write "NG code"(7) -> ()
                }
              }
            }
          }
        }
        frame #2 {
          n162 = local read "NG code"() -> (w363:dbl)
          n163 = Equal To 0?(x=w363) -> (x = 0?=w362:bool)
          n164 = case shown="True" w362 {
            tunnel: w364 -> [_ w365]
            frame False {
            }
            frame True {
              n165 = for {
                tunnel: w365 -> [w369] mode=indexing
                n166 = local read "glitch (mil)"() -> (w367:dbl)
                n167 = Unbundle By Name(w369) -> ("D_giltch"=w368:ext)
                n168 = Greater?(x=w368, y=w367) -> (0:w366:bool)
                n169 = case shown="True" w366 {
                  frame False {
                  }
                  frame True {
                    n170 = local write "NG code"(2) -> ()
                  }
                }
              }
            }
          }
        }
        frame #3 {
          n171 = local read "NG code"() -> (w373:dbl)
          n172 = Equal To 0?(x=w373) -> (x = 0?=w372:bool)
          n173 = case shown="True" w372 {
            tunnel: w371 -> [_ w374]
            frame False {
            }
            frame True {
              n174 = for {
                tunnel: w374 -> [w377] mode=indexing
                n175 = local read "damaged (mil)"() -> (w375:dbl)
                n176 = Unbundle By Name(w377) -> ("D_damaged"=w378:ext)
                n177 = Greater?(x=w378, y=w375) -> (0:w376:bool)
                n178 = case shown="True" w376 {
                  frame False {
                  }
                  frame True {
                    n179 = local write "NG code"(4) -> ()
                  }
                }
              }
            }
          }
        }
        frame #4 {
          n180 = local read "NG code"() -> (w382:dbl)
          n181 = Equal To 0?(x=w382) -> (x = 0?=w381:bool)
          n182 = case shown="True" w381 {
            tunnel: w380 -> [_ w400]
            frame False {
            }
            frame True {
              n183 = Index Array(array=w400, index=2) -> (element=w396:ext)
              n184 = Index Array(array=w400, index=3) -> (element=w394:ext)
              n185 = Index Array(array=w400, index=0) -> (element=w397:ext)
              n186 = Index Array(array=w400, index=1) -> (element=w395:ext)
              n187 = Divide(x=w397, y=w396) -> (x/y=w391:ext)
              n188 = Divide(x=w395, y=w394) -> (x/y=w388:ext)
              n189 = Decrement(x=w388) -> (x-1=w389:ext)
              n190 = Decrement(x=w391) -> (x-1=w393:ext)
              n191 = Greater Than 0?(x=w389) -> (x > 0?=w390:bool)
              n192 = Greater Than 0?(x=w393) -> (x > 0?=w392:bool)
              n193 = local read "ratio (cutting offest)"() -> (w383:dbl)
              n194 = case shown="True" w390 {
                tunnel: w388 -> [w405 w407]
                tunnel: [w405 w406] -> w385
                frame False {
                }
                frame True {
                  n195 = Reciprocal(x=w407) -> (1/x=w406:ext)
                }
              }
              n196 = case shown="True" w392 {
                tunnel: w391 -> [w408 w410]
                tunnel: [w408 w409] -> w387
                frame False {
                }
                frame True {
                  n197 = Reciprocal(x=w410) -> (1/x=w409:ext)
                }
              }
              n198 = Less?(x=w387, y=w383) -> (x < y?=w386:bool)
              n199 = Less?(x=w385, y=w383) -> (x < y?=w384:bool)
              n200 = case shown="True" w386 {
                frame False {
                }
                frame True {
                  n201 = local write "NG code"(5) -> ()
                }
              }
              n202 = case shown="True" w384 {
                frame False {
                }
                frame True {
                  n203 = local write "NG code"(5) -> ()
                }
              }
            }
          }
        }
        frame #5 {
          n204 = local read "NG code"() -> (w412:dbl)
          n205 = Equal To 0?(x=w412) -> (x = 0?=w411:bool)
          n206 = case shown="False" w411 {
            frame False {
            }
            frame True {
            }
          }
        }
        frame #6 {
          n207 = local read "NG code"() -> (w414:dbl)
          n208 = Equal To 0?(x=w414) -> (x = 0?=w413:bool)
          n209 = local write "PASS"(w413) -> ()
          n210 = Tick Count (ms)() -> (millisecond timer value=w417:u32)
          n211 = Subtract(x=w417, y=w416) -> (x-y=→"time image processing":u32)
        }
      }
    }
  }
